vi "Initialize RFSG.vi"(5 "Frequency Offset":i32=100, 6 "Selected Waveform":u16, 7 "Center Frequency":dbl, 8 "error in (no error)":errorcluster, 9 "IQ Rate":dbl, 10 "Power Level":dbl, 11 "RFSG Reference In":refnum<k15>) -> (0 "error out":errorcluster, 1 "Actual IQ Rate (S/s)":dbl, 2 "Frequecy Offset":dbl, 3 "RFSG Reference Out":refnum<k15>)   [LabVIEW 2021]
uses:
  <instrlib>/niRFSG/niRFSG.llb/niRFSG Write Arb Waveform (I-Q).vi
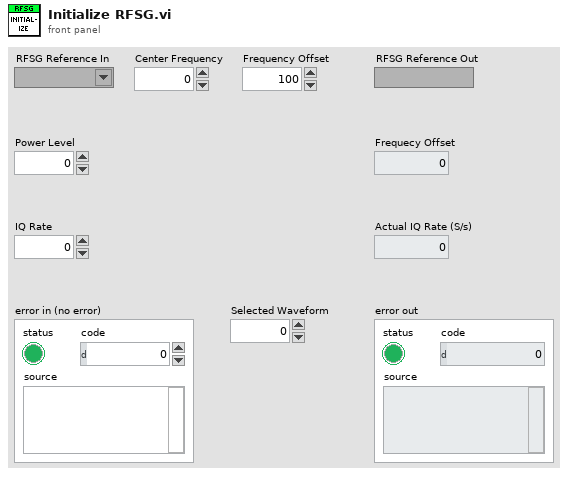
[diagram p1: front panel]
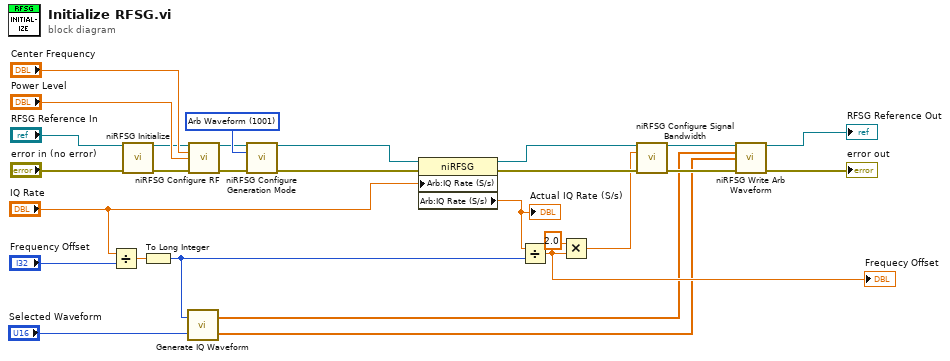
[diagram p0: block diagram]
diagram:
  w15 = 1001 items=["CW"=1000, "Arb Waveform"=1001, "Script"=1002] ("generation mode")
  n1 = Divide(x="IQ Rate", y="Frequency Offset") -> (x/y=w1:dbl)
  n2 = call <instrlib>:"niRFSG Initialize.vi"("resource name"="RFSG Reference In", "error in"="error in (no error)") -> ("instrument handle"=w11:refnum<k15>, "error out"=w12:errorcluster)  [unwired: 12 in]
  n3 = To Long Integer(number=w1) -> (32bit integer=w2:i32)
  n4 = call "Generate IQ Waveform.vi"("Selected Waveform"="Selected Waveform", "Samples Per Cycle"=w2) -> ("Q"=w8:dbl[], "I"=w9:dbl[])
  n5 = call <instrlib>:"niRFSG Configure RF.vi"("instrument handle"=w11, "frequency (Hz)"="Center Frequency", "power level (dBm)"="Power Level", "error in"=w12) -> ("instrument handle out"=w13:refnum<k15>, "error out"=w14:errorcluster)  [unwired: 10 in]
  n6 = call <instrlib>:"niRFSG Configure Generation Mode.vi"("instrument handle"=w13, "generation mode"=w15, "error in"=w14) -> ("instrument handle out"=w6:refnum<k15>, "error out"=w7:errorcluster)  [unwired: 11 in]
  n7 = property class="niRFSG"(reference=w6, error in=w7, "Arb:IQ Rate (S/s)"="IQ Rate") -> (reference out=w22:refnum<k15>, error out=w23:errorcluster, "Arb:IQ Rate (S/s)"=w16:dbl)
  "Actual IQ Rate (S/s)" <- w16
  n8 = Divide(x=w16, y=w2) -> (x/y=w24:dbl)
  "Frequecy Offset" <- w24
  n9 = Multiply(x=2.0 ("y"), y=w24) -> (x*y=w17:dbl)
  n10 = call <instrlib>:"niRFSG Configure Signal Bandwidth.vi"("instrument handle"=w22, "signal bandwidth (Hz)"=w17, "error in"=w23) -> ("instrument handle out"=w19:refnum<k15>, "error out"=w20:errorcluster)  [unwired: 11 in]
  n11 = call-poly <instrlib>:"niRFSG Write Arb Waveform.vi"("instrument handle"=w19, "I Data"=w9, "Q Data"=w8, "error in"=w20) -> ("instrument handle out"=→"RFSG Reference Out":refnum<k15>, "error out"=→"error out":errorcluster)  [unwired: 10 in]
